vi "Write Resultado.vi"(8 "error in (no error)":errorcluster, 10 "Resultado":dbl, 11 "Calculadora in":refnum<class "Calculadora.lvclass">) -> (0 "error out":errorcluster, 3 "Calculadora out":refnum<class "Calculadora.lvclass">)   [LabVIEW 2020, in "Calculadora.lvlib" / "Calculadora.lvclass"]
uses:
  Calculadora.lvclass
  Calculadora.lvclass/Calculadora.ctl
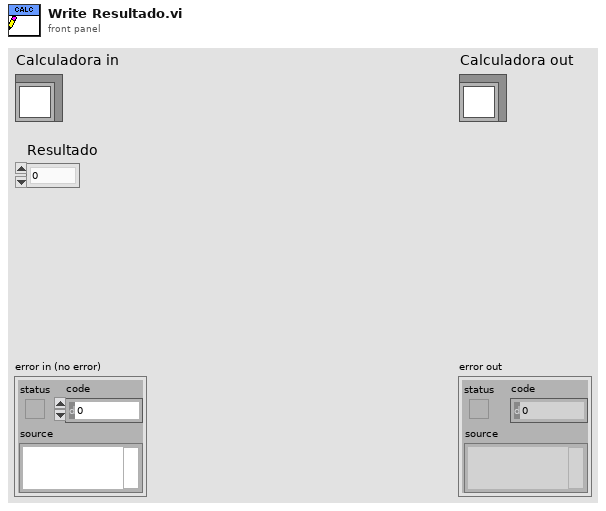
[diagram p1: front panel]
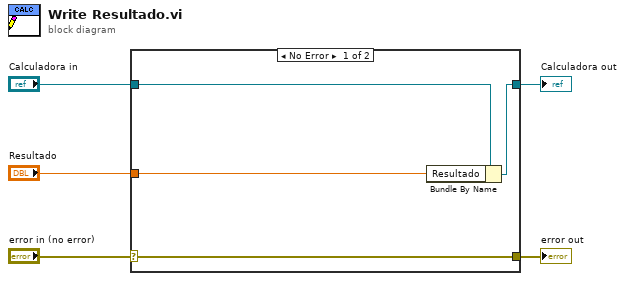
[diagram p0: block diagram]
diagram:
  n1 = case shown="No Error" "error in (no error)" {
    selector: "error in (no error)" -> [w9 w10]
    tunnel: [w9 w10] -> w4
    tunnel: [w7 w11] -> w2
    tunnel: "Calculadora in" -> [w8 w11]
    tunnel: "Resultado" -> [w6 _]
    frame No Error {
      n2 = Bundle By Name(cluster=w8, "Resultado"=w6) -> (w7:refnum<class "Calculadora.lvclass">)
    }
    frame Error {
    }
  }
  "error out" <- w4
  "Calculadora out" <- w2
